vi "Change Terminals to Non-Icon View.vi"(8 "error in":errorcluster, 11 "Folder Path":path) -> (0 "error out":errorcluster)   [LabVIEW 2020, in "PluginMetaDataObj.lvclass"]
doc: "This VI renames all the necessary classes and libraries to the custom name."
uses:
  PluginMetaDataObj.lvclass
  <vilib>/Utility/traverseref.llb/TRef TravTarget.ctl
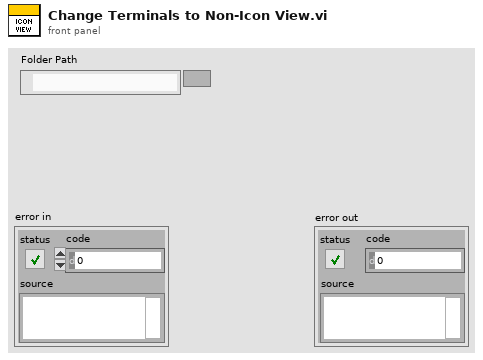
[diagram p1: front panel]
types:
  T1 = typedef "TRef TravTarget.ctl" = enum16{"FP", "BD", "Other"}
  T2 = enum32{"invalid VI type", "Standard VI", "Control VI", "Global VI", "Polymorphic VI", "Configuration VI", "SubSystem", "Facade VI", "Method VI", "Statechart Diagram VI"}
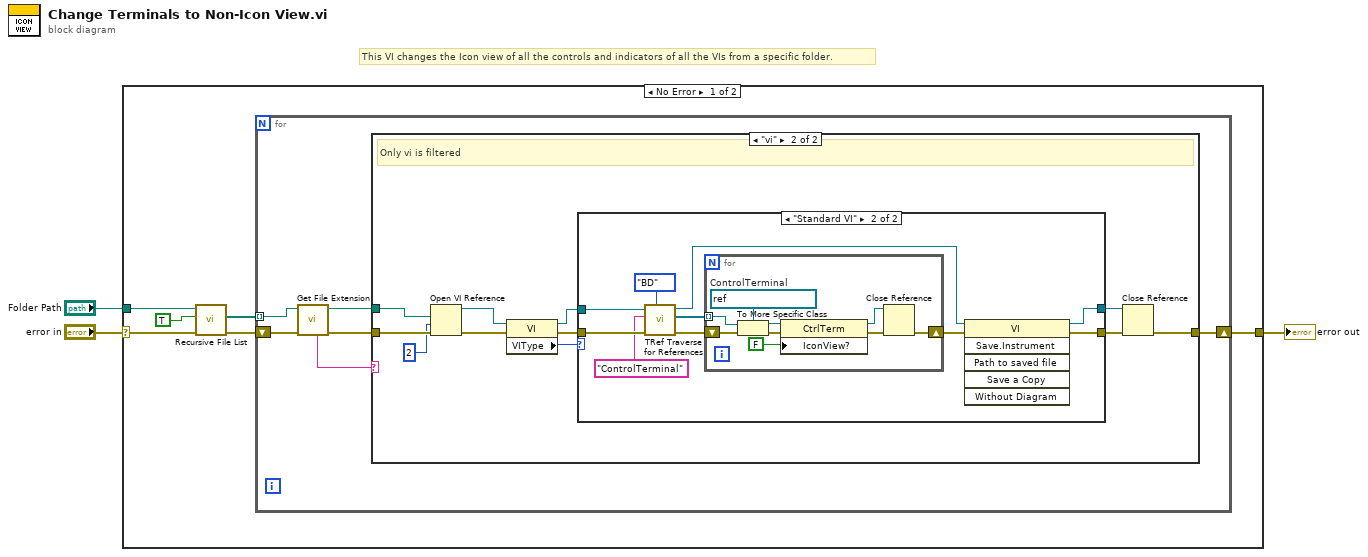
[diagram p0: block diagram]
diagram:
  # "This VI changes the Icon view of all the controls and indicators of all the VIs from a specific folder."
  n1 = case shown="No Error" "error in" {
    selector: "error in" -> [w7 w49]
    tunnel: [w6 w49] -> w2
    tunnel: "Folder Path" -> [w5 _]
    frame No Error {
      n2 = call <vilib>:"Recursive File List.vi"("error in (no error)"=w7, "Treat LLBs as Folders?"=TRUE, "Folder Path"=w5) -> ("error out"=w9:errorcluster, "All Files in Dir"=w8:path[])  [unwired: 4 in, 3 out]
      n3 = for {
        shift-right: [w15] -> w6
        shift-left: w9 -> [w13]
        tunnel: w8 -> [w14] mode=indexing
        n4 = call <vilib>:"Get File Extension.vi"("error in (no error)"=w13, "file"=w14) -> ("error out"=w12:errorcluster, "dup file"=w11:path, "unmodified file extension"=w10:string)  [unwired: 5 in, 2 out]
        n5 = case shown="\"vi\"" w10 {
          tunnel: w12 -> [w16 w25]
          tunnel: [w16 w24] -> w15
          tunnel: w11 -> [_ w22]
          frame "False", Default {
            # "No change in other type of file"
          }
          frame "vi" {
            # "Only vi is filtered"
            n6 = Open VI Reference(vi path=w22, options=2, error in (no error)=w25) -> (vi reference=w26:refnum<vi>, error out=w27:errorcluster)  [unwired: 3 in]
            n7 = property class="VI"(reference=w26, error in=w27) -> (reference out=w19:refnum<vi>, error out=w20:errorcluster, "VIType"=w21:T2)
            n8 = case shown="\"Standard VI\"" w21 {
              tunnel: w20 -> [w28 w39]
              tunnel: w19 -> [w29 w38]
              tunnel: [w29 w34] -> w18
              tunnel: [w28 w35] -> w17
              frame Default {
              }
              frame "Standard VI" {
                n9 = call <vilib>:"TRef Traverse for References.vi"("Traverse Target"=TRef_TravTarget."BD", "error in (no error)"=w39, "Class Name"="ControlTerminal", "VI Refnum"=w38) -> ("error out"=w32:errorcluster, "References"=w30:refnum<vi>[], "dup VI Refnum"=w33:refnum<vi>)  [unwired: 4 in, 1 out]
                n10 = for {
                  shift-right: [w43] -> w31
                  shift-left: w32 -> [w48]
                  tunnel: w30 -> [w47] mode=indexing
                  w46 = refnum<vi> refnum  # ControlTerminal
                  n11 = To More Specific Class(target class=w46, reference=w47, error in=w48) -> (specific class reference=w44:refnum<vi>, error out=w45:errorcluster)
                  n12 = property class="CtrlTerm"(reference=w44, error in=w45, "IconView?"=FALSE ("Icon View?")) -> (reference out=w41:refnum<vi>, error out=w42:errorcluster)
                  n13 = Close Reference(reference=w41, error in (no error)=w42) -> (error out=w43:errorcluster)
                }
                n14 = invoke class="VI" method="Save.Instrument"(reference=w33, error in=w31) -> (reference out=w34:refnum<vi>, error out=w35:errorcluster)  [unwired: 4 in, 4 out]
              }
            }
            n15 = Close Reference(reference=w18, error in (no error)=w17) -> (error out=w24:errorcluster)
          }
        }
      }
    }
    frame Error {
    }
  }
  "error out" <- w2
